vi "Handle Message.vi"(5 "Stack ID":u8, 7 "Function ID":u8, 8 "error in (no error)":errorcluster, 10 "Data":string, 11 "DC Brick in":refnum<class "DC Brick.lvclass">) -> (0 "error out":errorcluster, 1 "Send Answer":bool, 2 "Answer":variant, 3 "DC Brick out":refnum<class "DC Brick.lvclass">)   [LabVIEW 2011, in "Tinkerforge.lvlib" / "DC Brick.lvclass"]
doc: "This VI is the child implementation of \"Handle Message.vi\" and processes all responses for this device type."
uses:
  DC Brick.lvclass
  DC Brick.lvclass/DC Brick.ctl
  Device/Device.lvclass
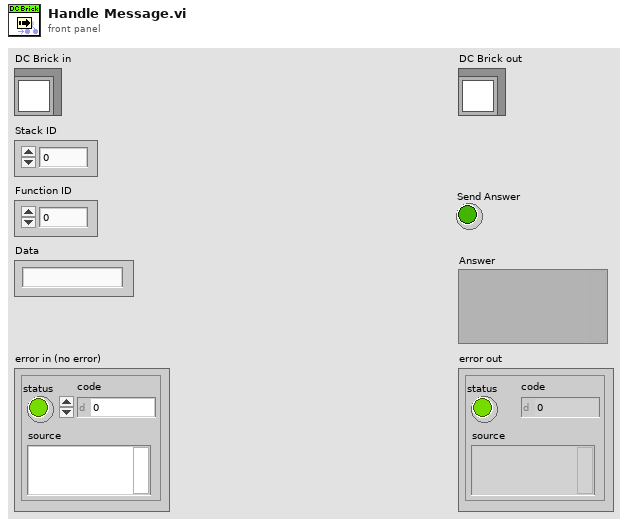
[diagram p1: front panel]
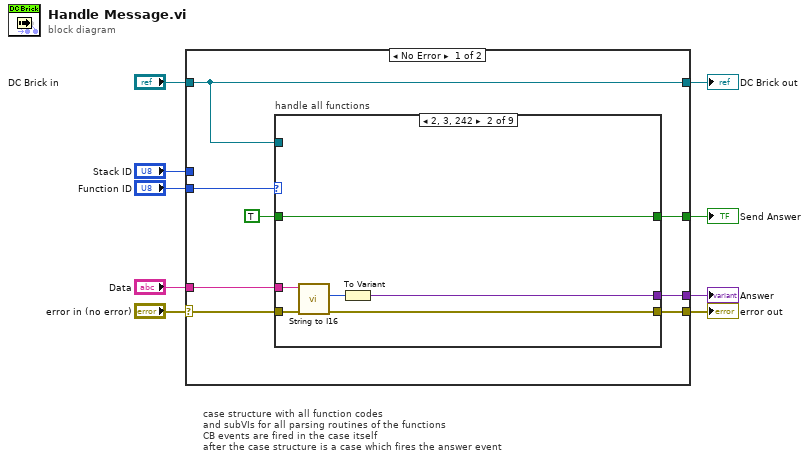
[diagram p0: block diagram]
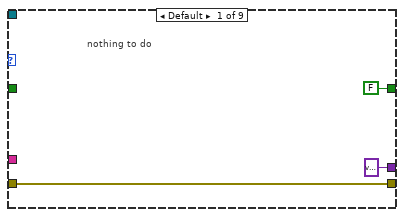
[diagram p2: hidden frame]
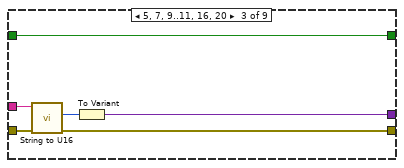
[diagram p3: hidden frame]
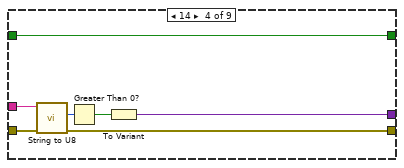
[diagram p4: hidden frame]
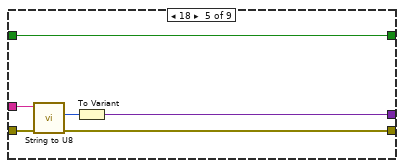
[diagram p5: hidden frame]
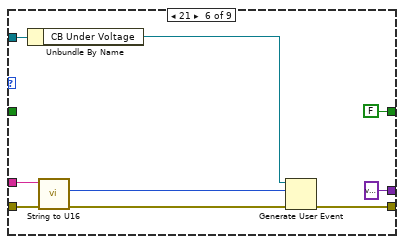
[diagram p6: hidden frame]
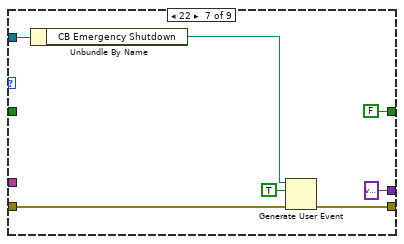
[diagram p7: hidden frame]
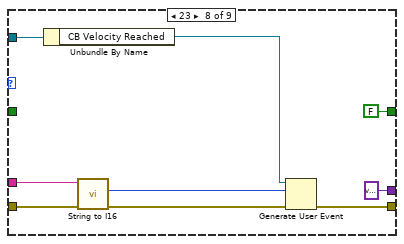
[diagram p8: hidden frame]
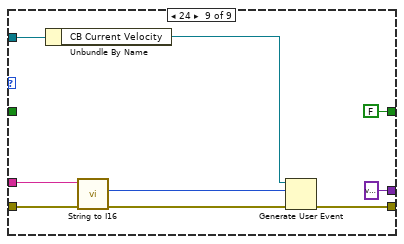
[diagram p9: hidden frame]
diagram:
  # "case structure with all function codes\nand subVIs for all parsing routines of the functions\nCB events are fired in the case itself\nafter the case structure is a case which fires the answer event"
  n1 = case shown="No Error" "error in (no error)" {
    selector: "error in (no error)" -> [w14 w80]
    tunnel: "DC Brick in" -> [w17 w81]
    tunnel: "Stack ID" -> [_ _]
    tunnel: "Function ID" -> [w16 _]
    tunnel: "Data" -> [w13 _]
    tunnel: [w17 w81] -> w4
    tunnel: [w12 w80] -> w3
    tunnel: [w11 _] -> w2
    tunnel: [w10 _] -> w1
    frame No Error {
      n2 = case "handle all functions" shown="2, 3, 242" w16 {
        tunnel: w14 -> [w20 w24 w31 w37 w43 w51 w56 w65 w74]
        tunnel: TRUE -> [_ w26 w32 w39 w45 _ _ _ _]
        tunnel: [FALSE w26 w32 w39 w45 FALSE FALSE FALSE FALSE] -> w10
        tunnel: [w20 w22 w30 w36 w40 w47 w57 w66 w75] -> w12
        tunnel: [variant ("Variant") w25 w27 w38 w44 variant ("Variant") variant ("Variant") variant ("Variant") variant ("Variant")] -> w11
        tunnel: w17 -> [_ _ _ _ _ w52 w59 w68 w77]
        tunnel: w13 -> [_ w23 w29 w35 w42 w50 _ w63 w72]
        frame Default {
          # "nothing to do"
        }
        frame 2, 3, 242 {
          n3 = call "String to I16.vi"("Error In"=w24, "String"=w23) -> ("Error Out"=w22:errorcluster, "I16"=w21:i16)  [unwired: 7 in, 1 out]
          n4 = To Variant(anything=w21) -> (Variant=w25:variant)
        }
        frame 5, 7, 9..11, 16, 20 {
          n5 = call "String to U16.vi"("Error In"=w31, "String"=w29) -> ("Error Out"=w30:errorcluster, "U16"=w28:u16)  [unwired: 7 in, 1 out]
          n6 = To Variant(anything=w28) -> (Variant=w27:variant)
        }
        frame 14 {
          n7 = call "String to U8.vi"("Error In"=w37, "String"=w35) -> ("Error Out"=w36:errorcluster, "U8"=w34:u8)  [unwired: 7 in, 1 out]
          n8 = Greater Than 0?(x=w34) -> (x > 0?=w33:bool)
          n9 = To Variant(anything=w33) -> (Variant=w38:variant)
        }
        frame 18 {
          n10 = call "String to U8.vi"("Error In"=w43, "String"=w42) -> ("Error Out"=w40:errorcluster, "U8"=w41:u8)  [unwired: 7 in, 1 out]
          n11 = To Variant(anything=w41) -> (Variant=w44:variant)
        }
        frame 21 {
          n12 = Unbundle By Name(w52) -> ("CB Under Voltage"=w48:refnum<user-event>)
          n13 = call "String to U16.vi"("Error In"=w51, "String"=w50) -> ("Error Out"=w49:errorcluster, "U16"=w46:u16)  [unwired: 7 in, 1 out]
          n14 = Generate User Event(user event=w48, event data cluster=w46, error in=w49) -> (error out=w47:errorcluster)  [unwired: 1 out]
        }
        frame 22 {
          n15 = Unbundle By Name(w59) -> ("CB Emergency Shutdown"=w58:refnum<user-event>)
          n16 = Generate User Event(user event=w58, event data cluster=TRUE ("event data"), error in=w56) -> (error out=w57:errorcluster)  [unwired: 1 out]
        }
        frame 23 {
          n17 = Unbundle By Name(w68) -> ("CB Velocity Reached"=w67:refnum<user-event>)
          n18 = call "String to I16.vi"("Error In"=w65, "String"=w63) -> ("Error Out"=w64:errorcluster, "I16"=w62:i16)  [unwired: 7 in, 1 out]
          n19 = Generate User Event(user event=w67, event data cluster=w62, error in=w64) -> (error out=w66:errorcluster)  [unwired: 1 out]
        }
        frame 24 {
          n20 = Unbundle By Name(w77) -> ("CB Current Velocity"=w76:refnum<user-event>)
          n21 = call "String to I16.vi"("Error In"=w74, "String"=w72) -> ("Error Out"=w73:errorcluster, "I16"=w71:i16)  [unwired: 7 in, 1 out]
          n22 = Generate User Event(user event=w76, event data cluster=w71, error in=w73) -> (error out=w75:errorcluster)  [unwired: 1 out]
        }
      }
    }
    frame Error {
    }
  }
  "error out" <- w3
  "DC Brick out" <- w4
  "Answer" <- w2
  "Send Answer" <- w1
